vi "Filtering.vi"(0 "Right border":sgl, 1 "Left border":sgl, 2 "Bottom border":sgl, 3 "fps":sgl, 4 "width":i32=5, 5 "height":i32=5) -> (7 "distance":sgl)   [LabVIEW 2020]
panel:
  out "lateral distance":sgl
  in  "length of mean average":i32=5
  out "relative acceleration":sgl
  out "relative speed":sgl
  out "moving average":sgl
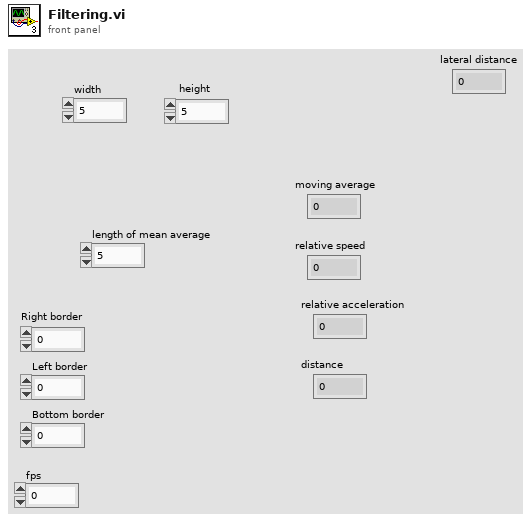
[diagram p1: front panel]
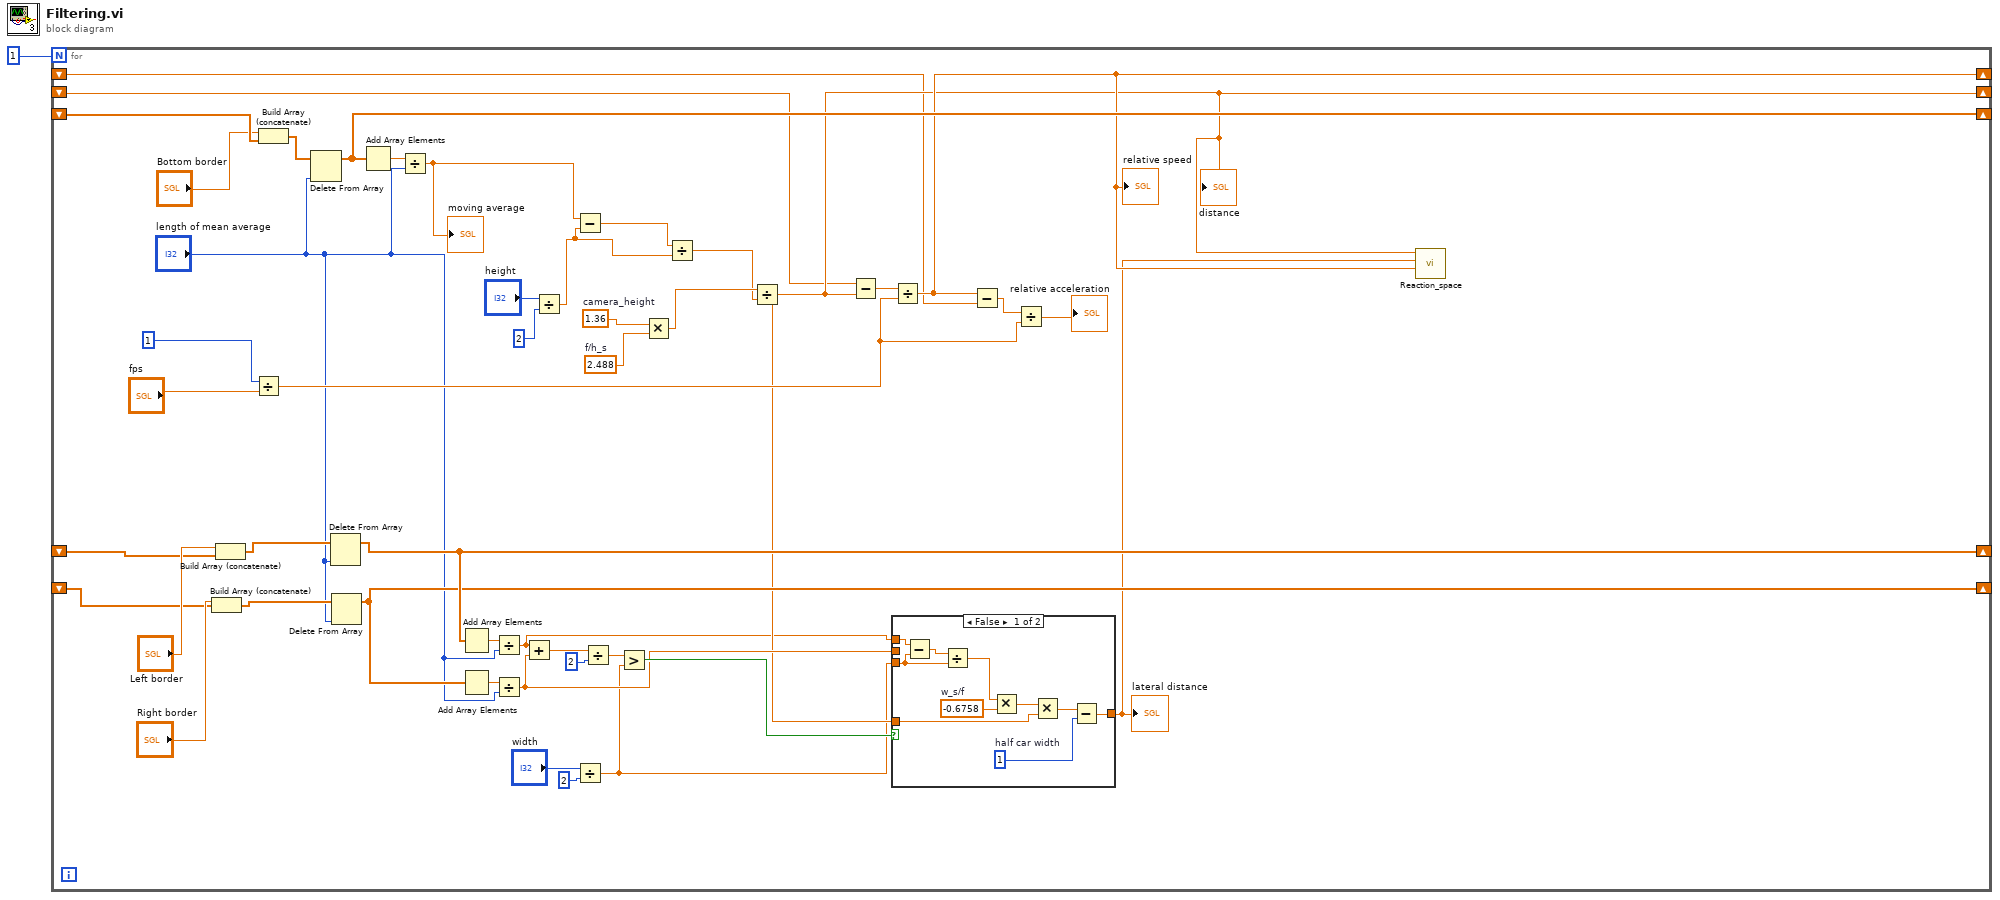
[diagram p0: block diagram]
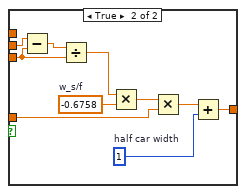
[diagram p2: hidden frame]
diagram:
  n1 = for {
    N: 1 -> [_]
    shift-right: [w20] -> _
    shift-left: _ -> [w11]
    shift-right: [w36] -> _
    shift-left: _ -> [w33]
    shift-right: [w14] -> _
    shift-left: _ -> [w10]
    shift-right: [w25] -> _
    shift-left: _ -> [w29]
    shift-right: [w24] -> _
    shift-left: _ -> [w28]
    w40 = 2.488  # f/h_s
    w39 = 1.36  # camera_height
    n2 = Build Array (concatenate)("Right border", w28) -> (w26:sgl[])
    n3 = Build Array (concatenate)("Left border", w29) -> (w27:sgl[])
    n4 = Divide(x=1, y="fps") -> (x/y=w44:sgl)
    n5 = Build Array (concatenate)("Bottom border", w33) -> (w35:sgl[])
    n6 = Delete From Array(array=w35, index="length of mean average") -> (array with subset deleted=w36:sgl[])  [unwired: 1 in, 1 out]
    n7 = Delete From Array(array=w27, index="length of mean average") -> (array with subset deleted=w25:sgl[])  [unwired: 1 in, 1 out]
    n8 = Delete From Array(array=w26, index="length of mean average") -> (array with subset deleted=w24:sgl[])  [unwired: 1 in, 1 out]
    n9 = Add Array Elements(numeric array=w36) -> (sum=w34:sgl)
    n10 = Divide(x=w34, y="length of mean average") -> (x/y=w37:sgl)
    "moving average" <- w37
    n11 = Add Array Elements(numeric array=w25) -> (sum=w23:sgl)
    n12 = Add Array Elements(numeric array=w24) -> (sum=w22:sgl)
    n13 = Divide(x=w23, y="length of mean average") -> (x/y=w13:sgl)
    n14 = Divide(x=w22, y="length of mean average") -> (x/y=w15:sgl)
    n15 = Add(x=w13, y=w15) -> (x+y=w19:sgl)
    n16 = Divide(x="height", y=2) -> (x/y=w2:dbl)
    n17 = Subtract(x=w37, y=w2) -> (x-y=w38:dbl)
    n18 = Divide(x="width", y=2) -> (x/y=w5:dbl)
    n19 = Divide(x=w19, y=2) -> (x/y=w17:sgl)
    n20 = Greater?(x=w17, y=w5) -> (0:w16:bool)
    n21 = Multiply(x=w39, y=w40) -> (x*y=w42:dbl)
    n22 = Divide(x=w38, y=w2) -> (x/y=w41:dbl)
    n23 = Divide(x=w42, y=w41) -> (x/y=w14:dbl)
    "distance" <- w14
    n24 = Subtract(x=w10, y=w14) -> (x-y=w43:dbl)
    n25 = case shown="False" w16 {
      tunnel: w15 -> [_ w66]
      tunnel: w5 -> [w48 w64]
      tunnel: w14 -> [w49 w60]
      tunnel: [w50 w57] -> w12
      tunnel: w13 -> [w47 _]
      frame False {
        w51 = 1  # half car width
        w52 = -0.6758  # w_s/f
        n26 = Subtract(x=w47, y=w48) -> (x-y=w53:dbl)
        n27 = Divide(x=w53, y=w48) -> (x/y=w54:dbl)
        n28 = Multiply(x=w54, y=w52) -> (x*y=w55:dbl)
        n29 = Multiply(x=w55, y=w49) -> (x*y=w56:dbl)
        n30 = Subtract(x=w56, y=w51) -> (x-y=w50:dbl)
      }
      frame True {
        w59 = 1  # half car width
        w62 = -0.6758  # w_s/f
        n31 = Subtract(x=w66, y=w64) -> (x-y=w65:dbl)
        n32 = Divide(x=w65, y=w64) -> (x/y=w63:dbl)
        n33 = Multiply(x=w63, y=w62) -> (x*y=w61:dbl)
        n34 = Multiply(x=w61, y=w60) -> (x*y=w58:dbl)
        n35 = Add(x=w58, y=w59) -> (x+y=w57:dbl)
      }
    }
    "lateral distance" <- w12
    n36 = Divide(x=w43, y=w44) -> (x/y=w20:dbl)
    "relative speed" <- w20
    n37 = Subtract(x=w20, y=w11) -> (x-y=w45:dbl)
    n38 = Divide(x=w45, y=w44) -> (x/y=→"relative acceleration":dbl)
    n39 = call "Reaction_space.vi"("Relative velocity m/s"=w20, "Obstacle Y"=w12, "Obstacle X"=w14) -> ()  [unwired: 9 in]
  }
